vi "C8855-01_Open.vi"(11 "MainD":T1 {"G_DIM" format="%.5f"}) -> (4 "Continue":bool, 15 "MainDR":T1 {"G_DIM" format="%.5f"})   [LabVIEW 2017]
uses:
  C8855_MainD.ctl
  C8855-01api.dll
panel:
  in  "H16":i32
  in  "H15":i32
  in  "H14":i32
  in  "H13":i32
  in  "H12":i32
  in  "H11":i32
  in  "H10":i32
  in  "H09":i32
  in  "H08":i32
  in  "H07":i32
  in  "H06":i32
  in  "H05":i32
  in  "H04":i32
  in  "H03":i32
  in  "H02":i32
  in  "H01":i32
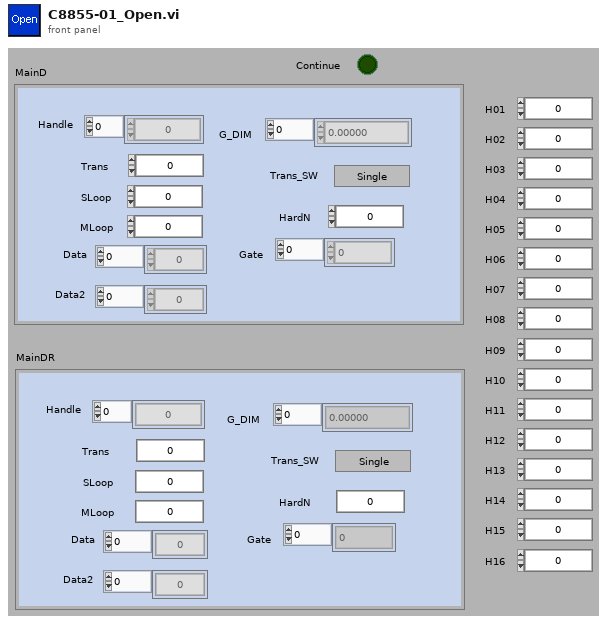
[diagram p1: front panel]
types:
  T1 = typedef "C8855_MainD.ctl" = cluster{"Handle":i32[], "G_DIM":dbl[], "Trans":u16, "Trans_SW":bool, "HardN":i32, "Gate":u8[], "Data":u32[], "Data2":u32[], "SLoop":i32, "MLoop":i32}
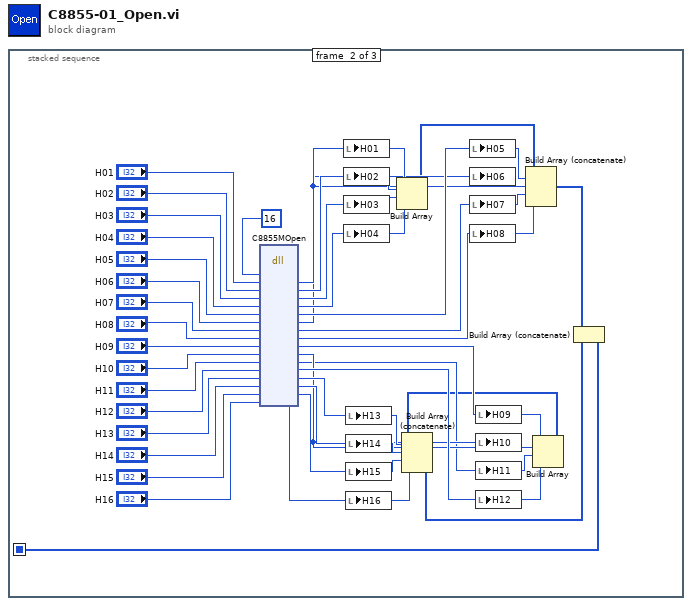
[diagram p0: block diagram]
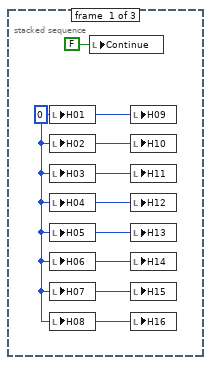
[diagram p2: hidden frame]
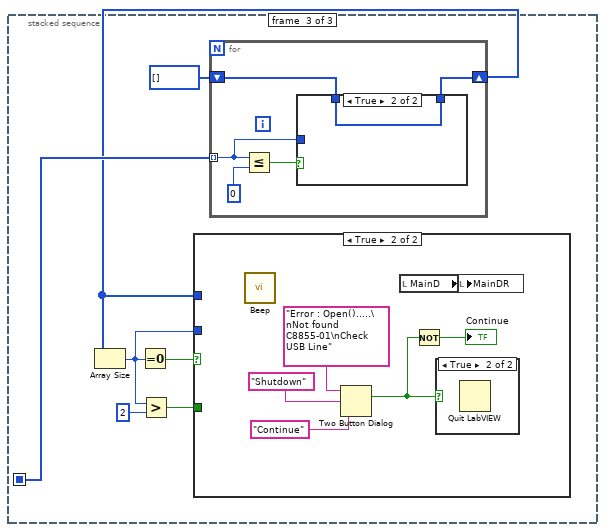
[diagram p3: hidden frame]
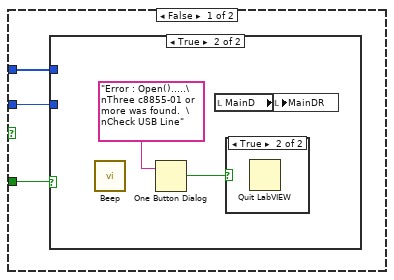
[diagram p4: hidden frame]
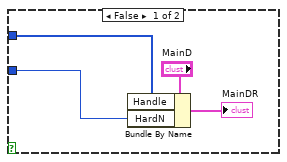
[diagram p5: hidden frame]
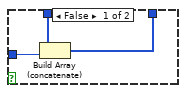
[diagram p8: hidden frame]
diagram:
  n1 = stacked-sequence {
    seq-local: [_ w3 _] -> [_ _ w47]
    frame #0 {
      w2 = 0 ("H01")
      n2 = local write "H01"(w2) -> ()
      n3 = local write "H02"(w2) -> ()
      n4 = local write "H03"(w2) -> ()
      n5 = local write "H04"(w2) -> ()
      n6 = local write "H05"(w2) -> ()
      n7 = local write "H06"(w2) -> ()
      n8 = local write "H07"(w2) -> ()
      n9 = local write "H08"(w2) -> ()
      n10 = local write "Continue"(FALSE ("Continue")) -> ()
      n11 = local write "H09"(w2) -> ()
      n12 = local write "H10"(w2) -> ()
      n13 = local write "H11"(w2) -> ()
      n14 = local write "H12"(w2) -> ()
      n15 = local write "H13"(w2) -> ()
      n16 = local write "H14"(w2) -> ()
      n17 = local write "H15"(w2) -> ()
      n18 = local write "H16"(w2) -> ()
    }
    frame #1 {
      n19 = dll-call lib="PTH2zabs CUsersPC33412Desktop\nkishi_DataC8855-01DevC8855-01 Ver3.3(仮) 2020SampleSourcex86C8855-01api.dll" fn="C8855MOpen"("Unit"=u8 16, "H1"="H01", "H2"="H02", "H3"="H03", "H4"="H04", "H5"="H05", "H6"="H06", "H7"="H07", "H8"="H08", "H9"="H09", "H10"="H10", "H11"="H11", "H12"="H12", "H13"="H13", "H14"="H14", "H15"="H15", "H16"="H16") -> ("H1"=w22:i32, "H2"=w21:i32, "H3"=w20:i32, "H4"=w23:i32, "H5"=w18:i32, "H6"=w17:i32, "H7"=w16:i32, "H8"=w19:i32, "H9"=w11:i32, "H10"=w9:i32, "H11"=w8:i32, "H12"=w10:i32, "H13"=w15:i32, "H14"=w13:i32, "H15"=w12:i32, "H16"=w14:i32)  [unwired: 4 in, 3 out]
      n20 = local write "H01"(w22) -> ()
      n21 = local write "H02"(w21) -> ()
      n22 = local write "H03"(w20) -> ()
      n23 = local write "H04"(w23) -> ()
      n24 = local write "H13"(w15) -> ()
      n25 = local write "H14"(w13) -> ()
      n26 = local write "H15"(w12) -> ()
      n27 = local write "H16"(w14) -> ()
      n28 = Build Array(w22, w21, w20, w23) -> (w7:i32[])
      n29 = local write "H05"(w18) -> ()
      n30 = local write "H06"(w17) -> ()
      n31 = local write "H07"(w16) -> ()
      n32 = local write "H08"(w19) -> ()
      n33 = local write "H09"(w11) -> ()
      n34 = local write "H10"(w9) -> ()
      n35 = local write "H11"(w8) -> ()
      n36 = local write "H12"(w10) -> ()
      n37 = Build Array (concatenate)(w7, w18, w17, w16, w19) -> (w4:i32[])
      n38 = Build Array(w11, w9, w8, w10) -> (w6:i32[])
      n39 = Build Array (concatenate)(w6, w15, w13, w12, w14) -> (w5:i32[])
      n40 = Build Array (concatenate)(w4, w5) -> (w3:i32[])
    }
    frame #2 {
      n41 = for {
        shift-right: [w64] -> w42
        shift-left: i32[] [] -> [w65]
        tunnel: w47 -> [w66] mode=indexing
        n42 = Less Or Equal?(x=w66, y=0) -> (x <= y?=w67:bool)
        n43 = case shown="TRUE" w67 {
          tunnel: w66 -> [w71 _]
          tunnel: w65 -> [w70 w72]
          tunnel: [w69 w72] -> w64
          frame False {
            n44 = Build Array (concatenate)(w70, w71) -> (w69:i32[])
          }
          frame True {
          }
        }
      }
      n45 = Array Size(array=w42) -> (size(s)=w41:i32)
      n46 = Equal To 0?(x=w41) -> (x = 0?=w45:bool)
      n47 = Greater?(x=w41, y=2) -> (0:w43:bool)
      n48 = case shown="TRUE" w45 {
        tunnel: w43 -> [w50 _]
        tunnel: w42 -> [w49 _]
        tunnel: w41 -> [w48 _]
        frame False {
          n49 = case shown="TRUE" w50 {
            tunnel: w49 -> [w52 _]
            tunnel: w48 -> [w51 _]
            frame False {
              n50 = Bundle By Name(cluster="MainD", "Handle"=w52, "HardN"=w51) -> (→"MainDR":T1)
            }
            frame True {
              n51 = call <vilib>:"Beep.vi"() -> ()  [unwired: 3 in, 9 out]
              n52 = One Button Dialog(message="Error : Open().....\nThree c8855-01 or more was found.  \nCheck USB Line" ("爷景嫁")) -> (true=w57:bool)  [unwired: 1 out]
              n53 = local read "MainD"() -> (w55:T1)
              n54 = case shown="TRUE" w57 {
                frame False {
                }
                frame True {
                  n55 = Quit LabVIEW() -> ()  [unwired: 1 out]
                }
              }
              n56 = local write "MainDR"(w55) -> ()
            }
          }
        }
        frame True {
          n57 = call <vilib>:"Beep.vi"() -> ()  [unwired: 3 in, 9 out]
          n58 = Two Button Dialog(message="Error : Open().....\nNot found C8855-01\nCheck USB Line" ("爷景嫁"), 1:"Continue" ("Fボタン名(\"キャンセル\")"), 2:"Shutdown" ("Tボタン名(\"OK\")")) -> (T button?=w60:bool)
          n59 = local read "MainD"() -> (w58:T1)
          n60 = Not(x=w60) -> (.not. x?=→"Continue":bool)
          n61 = case shown="TRUE" w60 {
            frame False {
            }
            frame True {
              n62 = Quit LabVIEW() -> ()  [unwired: 1 out]
            }
          }
          n63 = local write "MainDR"(w58) -> ()
        }
      }
    }
  }
